vi "Create Entity.vi"(6 "Library":bool, 7 "Project":string, 8 "error in (no error)":errorcluster, 9 "Container":string, 10 "Folder":path, 11 "Entity Name in":string) -> (0 "error out":errorcluster, 2 "New Entity Path":path, 3 "Entity Name":string)   [LabVIEW 2020, in "Conditum-Tools.lvlib" / "Entity Editor.lvclass"]
uses:
  Entity Editor.lvclass
  Entity Editor.lvclass/Entity Editor.ctl
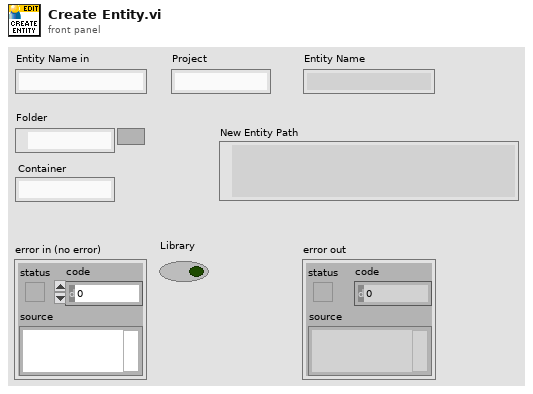
[diagram p1: front panel]
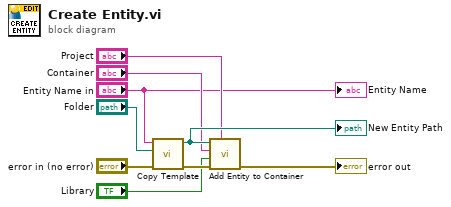
[diagram p0: block diagram]
diagram:
  n1 = call "Copy Template.vi"("error in (no error)"="error in (no error)", "Folder"="Folder", "Entity Name"="Entity Name in") -> ("error out"=w7:errorcluster, "New Library Path"=w6:path)  [unwired: 7 in]
  "New Entity Path" <- w6
  n2 = call "Add Entity to Container.vi"("Project"="Project", "error in (no error)"=w7, "Library"="Library", "Container"="Container", "Entity Path"=w6) -> ("error out"=→"error out":errorcluster)  [unwired: 5 in, 1 out]
  "Entity Name" <- "Entity Name in"
